vi "Unbenannt 1 (SubVI).vi"(11 "Cluster":T1) -> ()   [LabVIEW 2020]
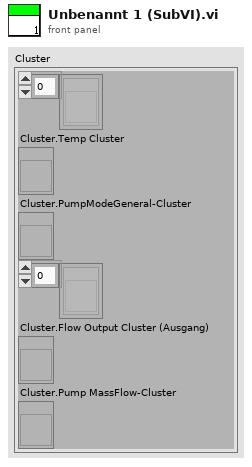
[diagram p1: front panel]
types:
  T1 = cluster{refnum<vi>[], "Cluster.Temp Cluster":refnum<vi>, "Cluster.PumpModeGeneral-Cluster":refnum<vi>, refnum<vi>[], "Cluster.Flow Output Cluster (Ausgang)":refnum<vi>, "Cluster.Pump MassFlow-Cluster":refnum<vi>}
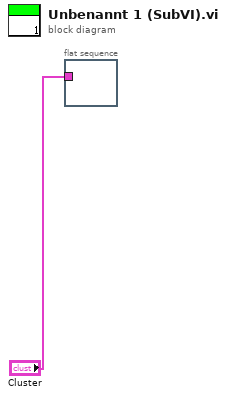
[diagram p0: block diagram]
diagram:
  n1 = flat-sequence {
    tunnel: "Cluster" -> [_]
    frame #0 {
    }
  }
